vi "BRig_RT__Case_Exp__State_initTrial2__Laser_Reward__v2.vi"(0 "input_L_OnOff":u16, 1 "input_L_Block":u16, 2 "input_L_Trial":u16, 3 "input_L_Probability":u16, 4 "input_L_nRew1":u16, 5 "input_L_nRew2":u16, 6 "input_nReward":u16, 8 "input_iSpout":u16, 10 "input_sState_start":u16, 12 "input_LaserSwitch":bool) -> (16 "output_LR_Event":bool, 17 "output_LR_Event_num":u16, 18 "output_LR_Laser":bool, 19 "output_LR_Laser_num":u16)   [LabVIEW 2014]
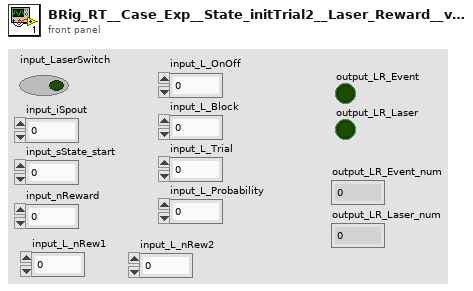
[diagram p1: front panel]
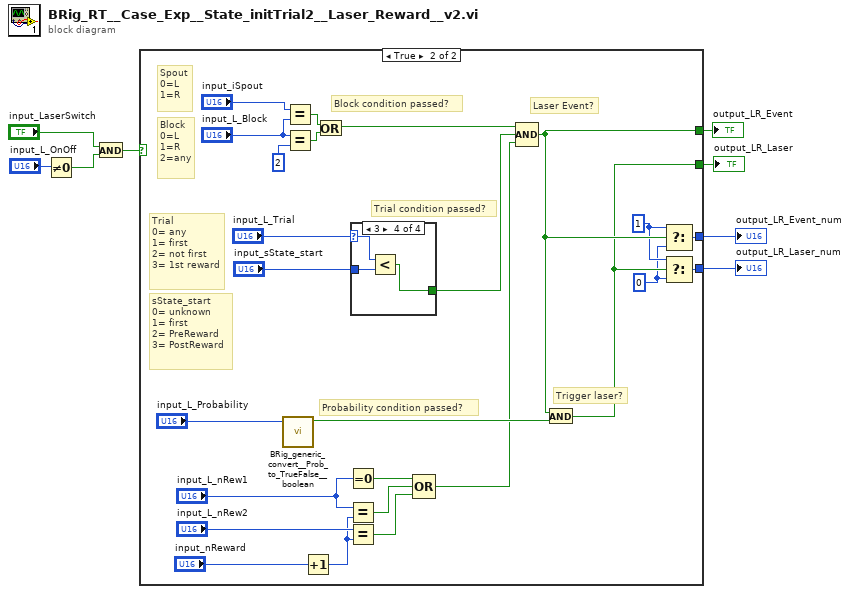
[diagram p0: block diagram]
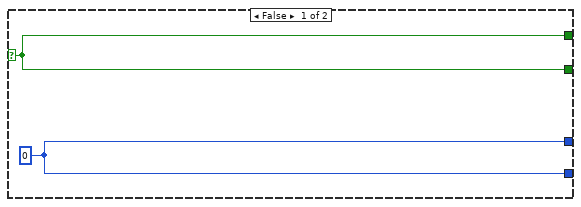
[diagram p2: hidden frame]
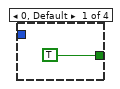
[diagram p3: hidden frame]
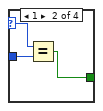
[diagram p4: hidden frame]
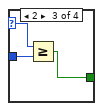
[diagram p5: hidden frame]
diagram:
  n1 = Not Equal To 0?(x="input_L_OnOff") -> (x != 0?=w7:bool)
  n2 = And(x="input_LaserSwitch", y=w7) -> (x .and. y?=w5:bool)
  n3 = case shown="True" w5 {
    selector: w5 -> [w10 _]
    tunnel: [w10 w24] -> w4
    tunnel: [w10 w23] -> w3
    tunnel: [w9 w20] -> w2
    tunnel: [w9 w19] -> w1
    frame False {
      w9 = u16 0 ("y")
    }
    frame True {
      w21 = u16 0 ("y")
      w22 = u16 1 ("y")
      # "Trigger laser?"
      # "Laser Event?"
      # "Trial condition passed?"
      # "sState_start\n0= unknown\n1= first\n2= PreReward\n3= PostReward"
      # "Probability condition passed?"
      # "Trial\n0= any\n1= first\n2= not first\n3= 1st reward"
      # "Block condition passed?"
      # "Spout\n0=L\n1=R"
      # "Block\n0=L\n1=R\n2=any"
      n4 = call "BRig_generic_convert__Prob_to_TrueFalse__boolean.vi"("input_probability_u16"="input_L_Probability") -> ("output_TF"=w25:bool)  [unwired: 10 in]
      n5 = Equal?(x="input_iSpout", y="input_L_Block") -> (x = y?=w35:bool)
      n6 = Equal?(x="input_L_Block", y=u16 2) -> (x = y?=w34:bool)
      n7 = Increment(x="input_nReward") -> (x+1=w13:u16)
      n8 = Or(x=w35, y=w34) -> (x .or. y?=w27:bool)
      n9 = Equal To 0?(x="input_L_nRew1") -> (x = 0?=w18:bool)
      n10 = Equal?(x="input_L_nRew1", y=w13) -> (x = y?=w12:bool)
      n11 = Equal?(x="input_L_nRew2", y=w13) -> (x = y?=w11:bool)
      n12 = case shown="3" "input_L_Trial" {
        selector: "input_L_Trial" -> [_ w38 w41 w44]
        tunnel: [TRUE w37 w40 w43] -> w26
        tunnel: "input_sState_start" -> [_ w39 w42 w45]
        frame 0, Default {
        }
        frame 1 {
          n13 = Equal?(x=w38, y=w39) -> (x = y?=w37:bool)
        }
        frame 2 {
          n14 = Greater Or Equal?(x=w41, y=w42) -> (x >= y?=w40:bool)
        }
        frame 3 {
          n15 = Less?(x=w44, y=w45) -> (x < y?=w43:bool)
        }
      }
      n16 = Compound Arithmetic op=OR(w18, w12, w11) -> (w17:bool)
      n17 = Compound Arithmetic op=AND(w27, w26, w17) -> (w24:bool)
      n18 = And(x=w24, y=w25) -> (x .and. y?=w23:bool)
      n19 = Select(t=w22, s=w24, f=w21) -> (s? t:f=w20:u16)
      n20 = Select(t=w22, s=w23, f=w21) -> (s? t:f=w19:u16)
    }
  }
  "output_LR_Event" <- w4
  "output_LR_Laser" <- w3
  "output_LR_Event_num" <- w2
  "output_LR_Laser_num" <- w1
